vi "Get Measurements.vi"(0 "object in":refnum<class "HPS-17000-PowerModule.lvclass">, 11 "Error In":errorcluster) -> (4 "object out":refnum<class "HPS-17000-PowerModule.lvclass">, 6 "measurements":T1[](array[typedef]), 15 "Error Out":errorcluster)   [LabVIEW 2023, in "HPS-17000-PowerModule.lvlib" / "HPS-17000-PowerModule.lvclass"]
uses:
  HPS-17000-PowerModule.lvclass
  builds/PowerModuleInterface/PowerModuleInterface.lvlibp/Classes/PowerModule_interface/Measurements.ctl
  HPS-17000-PowerModule.lvclass/HPS-17000-PowerModule.ctl
  builds/PowerModuleInterface/PowerModuleInterface.lvlibp/Classes/PowerModule_interface/PowerModuleInterface.lvclass
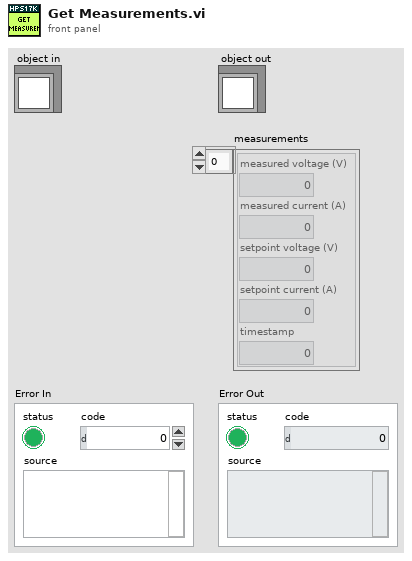
[diagram p1: front panel]
types:
  T1 = typedef "PowerModuleInterface.lvlibp/PowerModuleInterface.lvclass/Measurements.ctl" = cluster{"measured voltage (V)":dbl, "measured current (A)":dbl, "setpoint voltage (V)":dbl, "setpoint current (A)":dbl, "timestamp":dbl}
  T2 = typedef "HPS-17000-PowerModule.lvlib/HPS-17000-PowerModule.lvclass/ObjectAttributes.ctl" = cluster{"JSON Config Path":path, "Configuration":T3, "GM ID":string, "HPS17000 Refs":refnum<class "HPS-17000.lvclass">[], "connected":bool, "reserved":bool, "events":T5, "nibatterycycler_grpc_Setpoint":T6, "last timestamp":i64, "mode":T7, "range":T8, "measurement array":T1[], "measurement stream":bool, "setpoint stream":bool}
  T3 = typedef "HPS-17000-PowerModule.lvlib/HPS-17000-PowerModule.lvclass/Configuration.ctl" = cluster{"TSN NIC IP Address":string, "HPS17000 IP Addresses":string[], "HPS Topology":enum16{"SINGLE", "MULTI"}, "Setpoint Stream Config":T4, "Measurement Array Size":i32}
  T4 = typedef "Cycler.lvclass/Setpoint Stream Basic Config.ctl" = cluster{"local address":string, "receiver port":u16}
  T5 = typedef "HPS-17000.lvclass/Multi-Cycler Events.ctl" = cluster{"heartbeats events":refnum<user-event>[], "faults events":refnum<user-event>[], "network sync event":refnum<user-event>[], "setpoint status event":refnum<user-event>[]}
  T6 = typedef "NI_BC_client.lvlib/nibatterycycler_grpc_Setpoint.ctl" = cluster{"voltage":sgl, "current":sgl, "min_power":sgl, "max_power":sgl, "resistance":sgl}
  T7 = typedef "HPS-17000-PowerModule.lvlib/HPS-17000-PowerModule.lvclass/Mode.ctl" = u16
  T8 = typedef "PowerModuleInterface.lvlibp/PowerModuleInterface.lvclass/Range.ctl" = cluster{"Current Max (A)":dbl, "Current Min (A)":dbl, "Voltage Max (V)":dbl, "Voltage Min (V)":dbl}
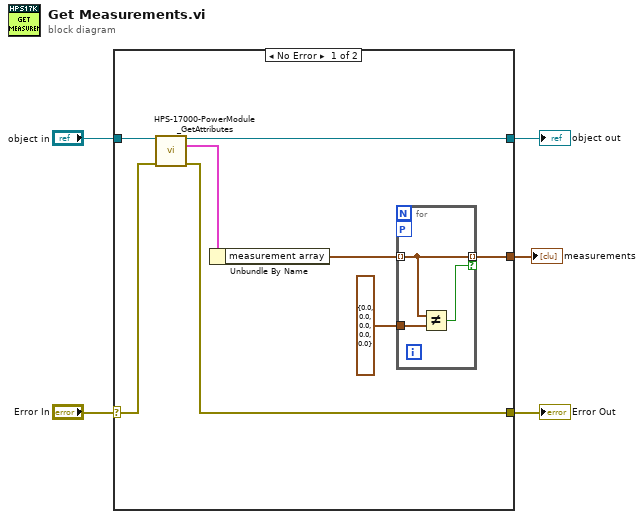
[diagram p0: block diagram]
diagram:
  n1 = case shown="No Error" "Error In" {
    selector: "Error In" -> [w12 w17]
    tunnel: "object in" -> [w13 w18]
    tunnel: [w10 w18] -> w5
    tunnel: [w11 w17] -> w2
    tunnel: [w6 _] -> w1
    frame No Error {
      n2 = call "HPS-17000-PowerModule_GetAttributes.vi"("reference in"=w13, "Error In"=w12) -> ("reference out"=w10:refnum<class "HPS-17000-PowerModule.lvclass">, "Data"=w9:T2, "Error Out"=w11:errorcluster)  [unwired: 10 in, 1 out]
      n3 = Unbundle By Name(w9) -> ("measurement array"=w8:T1[])
      n4 = for {
        tunnel: w8 -> [w15] mode=indexing
        workers-P: _ -> [_]
        tunnel: T1 {"measured voltage (V)"=0.0, "measured current (A)"=0.0, "setpoint voltage (V)"=0.0, "setpoint current (A)"=0.0, "timestamp"=0.0} ("Measurements") -> [w16]
        tunnel: [w15] -> w6 mode=indexing if=w14
        n5 = Not Equal?(x=w15, y=w16) -> (x != y?=w14:bool)
      }
    }
    frame Error {
    }
  }
  "Error Out" <- w2
  "object out" <- w5
  "measurements" <- w1
